vi "Read ADU Packet.vi"(8 "error in":errorcluster, 10 "isMaster (f)":bool, 11 "ELAN data unit (ADU) in":refnum<class "ELAN Data Unit.lvclass">) -> (0 "error out":errorcluster, 1 "ELAN data unit (PDU)":refnum<class "ELAN PDU.lvclass">, 3 "ELAN data unit (ADU) out":refnum<class "ELAN Data Unit.lvclass">, 5 "PDU Valid?":bool)   [LabVIEW 2021, in "ELAN Data Unit.lvclass"]
uses:
  ELAN Data Unit.lvclass
  Data Unit/ELAN PC Data Unit/ELAN PDU.lvclass
  ELAN Data Unit.lvclass/ELAN Data Unit.ctl
  Data Unit/ELAN PC Data Unit/ELAN PDU.lvclass/ELAN PDU.ctl
  Calculate CRC.vi
  <vilib>/ErrorRing/Error Ring.xnode
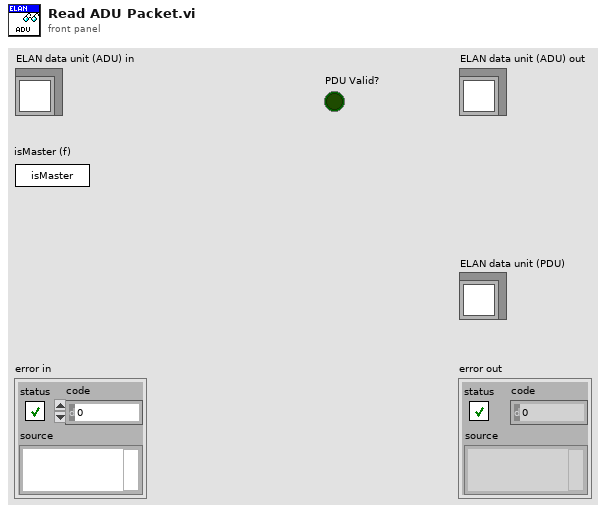
[diagram p1: front panel]
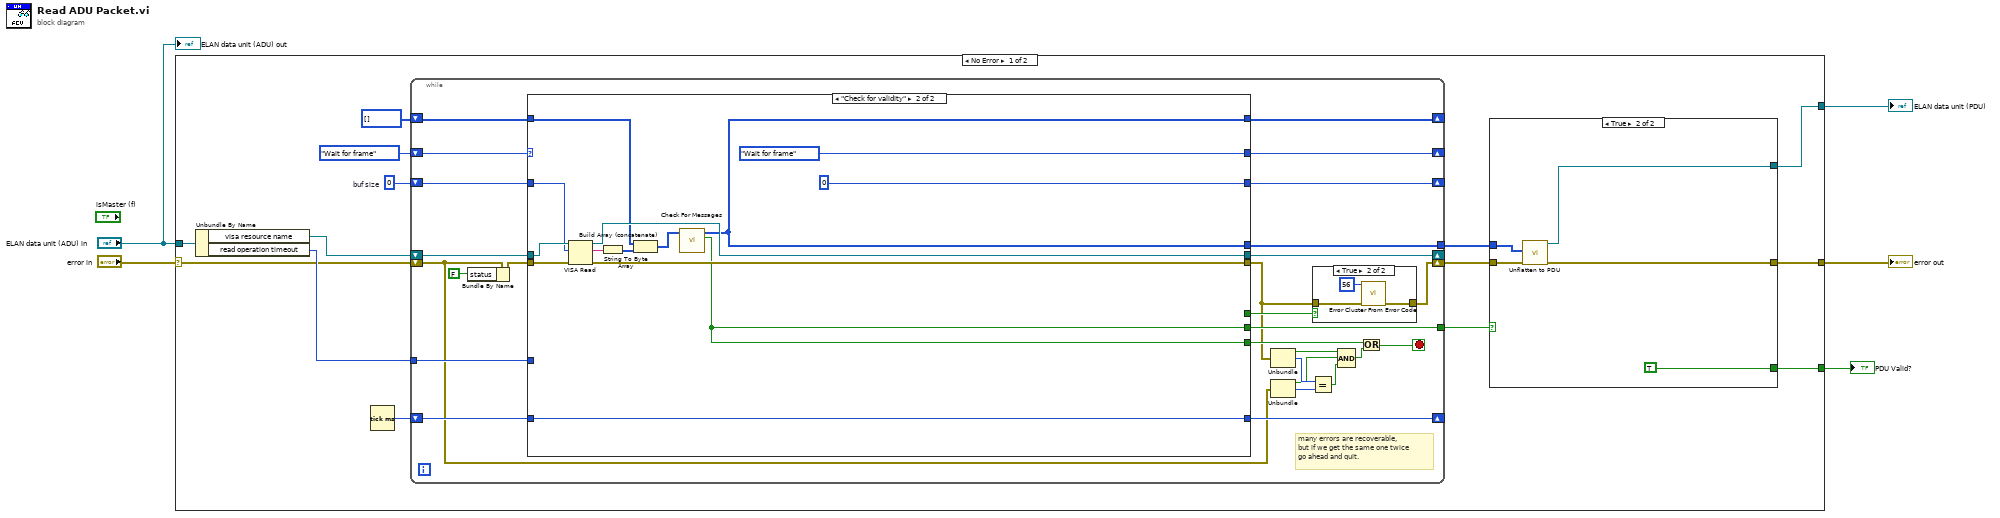
[diagram p0: block diagram]
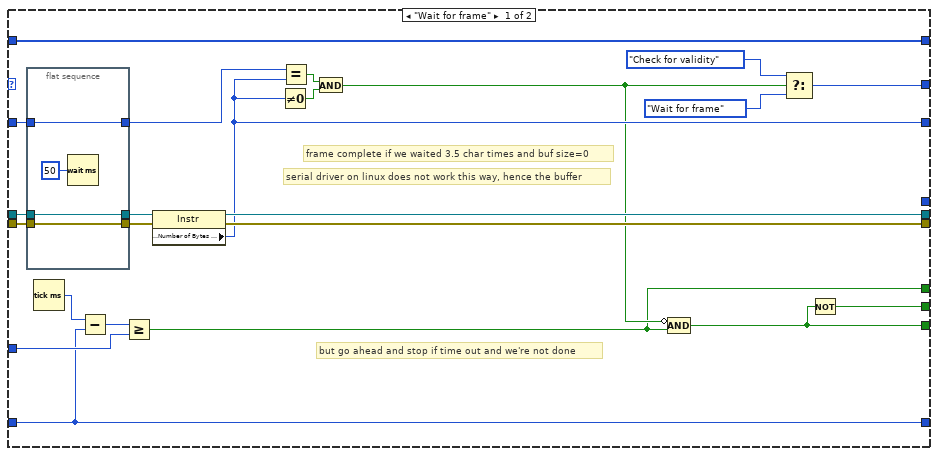
[diagram p3: hidden frame]
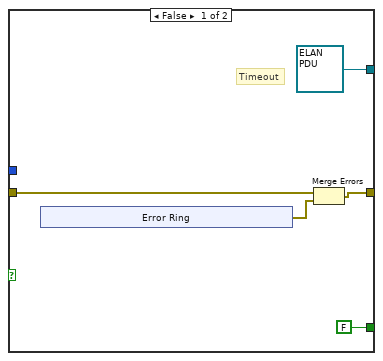
[diagram p4: hidden frame]
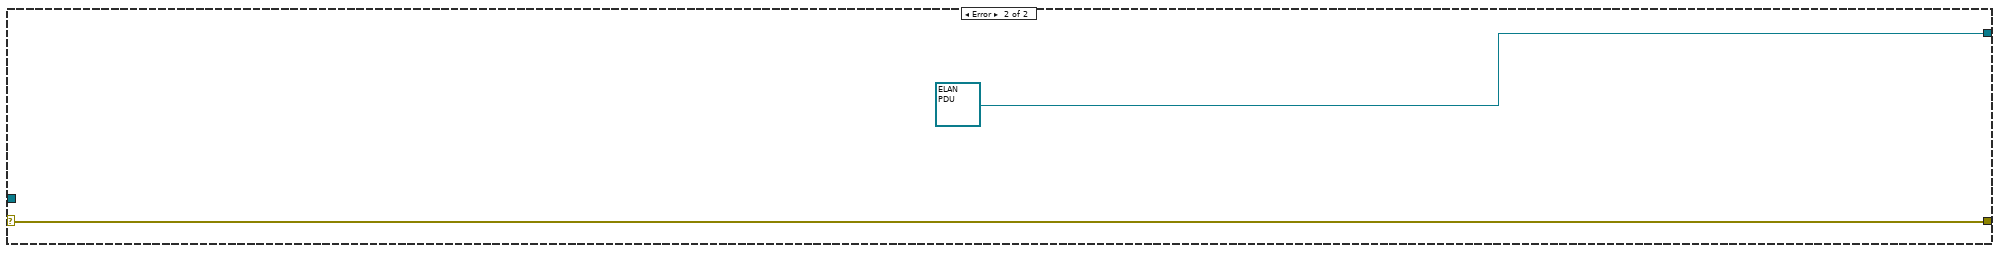
[diagram p5: hidden frame]
diagram:
  n1 = case shown="No Error" "error in" {
    selector: "error in" -> [w6 w107]
    tunnel: [w19 w107] -> w4
    tunnel: "ELAN data unit (ADU) in" -> [w16 _]
    tunnel: [w18 refnum<class "ELAN PDU.lvclass"> refnum ("modbus data unit")] -> w5
    tunnel: [w17 _] -> w3
    frame No Error {
      w11 = u32 0  # buf size
      n2 = Unbundle By Name(w16) -> ("visa resource name"=w15:refnum<visa-resource-name>, "read operation timeout"=w14:u32)
      n3 = Tick Count (ms)() -> (millisecond timer value=w13:u32)
      n4 = while {
        shift-right: [w35] -> w9
        shift-left: w6 -> [w26]
        shift-right: [w40] -> _
        shift-left: w15 -> [w45]
        shift-right: [w39] -> _
        shift-left: enum16{"Wait for frame", "Check for validity"}."Wait for frame" ("Serial Acquisition States") -> [w46]
        shift-right: [w41] -> _
        shift-left: w11 -> [w42]
        tunnel: w14 -> [w43]
        tunnel: [w38] -> w8
        tunnel: [w37] -> w7
        shift-right: [w33] -> _
        shift-left: u8[] [] -> [w34]
        shift-right: [w32] -> _
        shift-left: w13 -> [w44]
        stop <- w29 stop-if-true
        # "many errors are recoverable,\nbut if we get the same one twice\ngo ahead and quit."
        n5 = Bundle By Name(cluster=w26, "status"=FALSE) -> (w31:errorcluster)
        n6 = case shown="\"Check for validity\"" w46 {
          tunnel: w45 -> [w69 w90]
          tunnel: w31 -> [w68 w91]
          tunnel: w44 -> [w53 w79]
          tunnel: w43 -> [w71 _]
          tunnel: w42 -> [w66 w89]
          tunnel: [w59 u32 0 ("Bytes at Port")] -> w41
          tunnel: [w56 w80] -> w28
          tunnel: [w62 w81] -> w27
          tunnel: [w61 w88] -> w40
          tunnel: [w60 enum16{"Wait for frame", "Check for validity"}."Wait for frame" ("Serial Acquisition States")] -> w39
          tunnel: [w57 w80] -> w38
          tunnel: [_ w78] -> w37
          tunnel: [w55 _] -> w36
          tunnel: w34 -> [w54 w84]
          tunnel: [w54 w78] -> w33
          tunnel: [w53 w79] -> w32
          frame "Wait for frame" {
            # "serial driver on linux does not work this way, hence the buffer"
            # "but go ahead and stop if time out and we're not done"
            # "frame complete if we waited 3.5 char times and buf size=0"
            n7 = flat-sequence {
              tunnel: [w77] -> w70
              tunnel: w69 -> [w77]
              tunnel: w68 -> [w76]
              tunnel: [w76] -> w67
              tunnel: w66 -> [w75]
              tunnel: [w75] -> w63
              frame #0 {
                n8 = Wait (ms)(milliseconds to wait=u32 50 ("millisecond multiple")) -> ()  [unwired: 1 out]
              }
            }
            n9 = Tick Count (ms)() -> (millisecond timer value=w73:u32)
            n10 = Subtract(x=w73, y=w53) -> (x-y=w72:u32)
            n11 = Greater Or Equal?(x=w72, y=w71) -> (x >= y?=w55:bool)
            n12 = property class="Instr"(reference=w70, error in=w67) -> (reference out=w61:refnum<visa-resource-name>, error out=w62:errorcluster, "Serial Settings:Number of Bytes at Serial Port"=w59:u32)
            n13 = Not Equal To 0?(x=w59) -> (x != 0?=w65:bool)
            n14 = Equal?(x=w63, y=w59) -> (x = y?=w64:bool)
            n15 = And(x=w64, y=w65) -> (x .and. y?=w58:bool)
            n16 = Compound Arithmetic op=AND(invert w58, w55) -> (w56:bool)
            n17 = Select(t=enum16{"Wait for frame", "Check for validity"}."Check for validity" ("Serial Acquisition States"), s=w58, f=enum16{"Wait for frame", "Check for validity"}."Wait for frame" ("Serial Acquisition States")) -> (s? t:f=w60:enum16{"Wait for frame", "Check for validity"})
            n18 = Not(x=w56) -> (.not. x?=w57:bool)
          }
          frame "Check for validity" {
            n19 = VISA Read(VISA resource name=w90, byte count=w89, error in (no error)=w91) -> (VISA resource name out=w88:refnum<visa-resource-name>, read buffer=w85:string, error out=w81:errorcluster)  [unwired: 1 out]
            n20 = String To Byte Array(string=w85) -> (unsigned byte array=w83:u8[])
            n21 = Build Array (concatenate)(w84, w83) -> (w82:u8[])
            n22 = call "Check For Messages.vi"("data in"=w82) -> ("PDU valid?"=w80:bool, "data"=w78:u8[])  [unwired: 9 in]
          }
        }
        n23 = Unbundle(w27) -> ("status"=w23:bool, "code"=w24:i32)  [unwired: 1 out]
        n24 = Unbundle(w26) -> ("status"=w22:bool, "code"=w25:i32)  [unwired: 1 out]
        n25 = Equal?(x=w24, y=w25) -> (x = y?=w20:bool)
        n26 = case shown="True" w36 {
          tunnel: w27 -> [w47 w50]
          tunnel: [w47 w49] -> w35
          frame False {
          }
          frame True {
            n27 = call <vilib>:"Error Cluster From Error Code.vi"("error in (no error)"=w50, "error code (0)"=56) -> ("error out"=w49:errorcluster)  [unwired: 7 in]
          }
        }
        n28 = Compound Arithmetic op=AND(w23, w22, w20) -> (w21:bool)
        n29 = Or(x=w28, y=w21) -> (x .or. y?=w29:bool)
      }
      n30 = case shown="True" w8 {
        tunnel: w9 -> [w94 w103]
        tunnel: [refnum<class "ELAN PDU.lvclass"> refnum ("modbus data unit") w101] -> w18
        tunnel: [w93 w102] -> w19
        tunnel: [FALSE TRUE] -> w17
        tunnel: w7 -> [_ w104]
        frame False {
          # "Timeout"
          n31 = xnode "Error Ring"() -> ("error out"=w95:errorcluster)
          n32 = Merge Errors(w94, w95) -> (w93:errorcluster)
        }
        frame True {
          n33 = call "Unflatten to PDU.vi"("error in"=w103, "ELAN data unit data"=w104) -> ("error out"=w102:errorcluster, "ELAN data unit out"=w101:refnum<class "ELAN PDU.lvclass">)  [unwired: 8 in]
        }
      }
    }
    frame Error {
    }
  }
  "ELAN data unit (PDU)" <- w5
  "error out" <- w4
  "PDU Valid?" <- w3
  "ELAN data unit (ADU) out" <- "ELAN data unit (ADU) in"
